vi "SimpleGit-Settings.vi"(11 "path":path) -> ()   [LabVIEW 2017]
uses:
  <vilib>/Hampel Software Engineering/Git API/Git API/GIT-api.lvclass
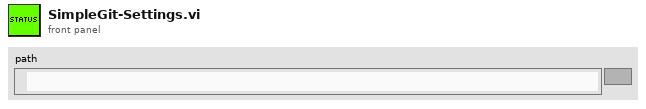
[diagram p1: front panel]
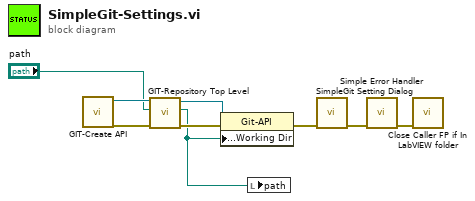
[diagram p0: block diagram]
diagram:
  n1 = call <vilib>:"GIT-Create API.vi"() -> ("error out"=w6:errorcluster, "git-api out"=w7:refnum<class "GIT-api.lvclass">)  [unwired: 10 in]
  n2 = call <vilib>:"GIT-Repository Top Level.vi"("error in"=w6, "Current Path"="path", "git-api in"=w7) -> ("error out"=w9:errorcluster, "Repo Top Level Path"=w3:path, "git-api out"=w8:refnum<class "GIT-api.lvclass">)  [unwired: 6 in]
  n3 = property class="Git-API"(reference=w8, error in=w9, "Accessors:Working Dir"=w3) -> (error out=w2:errorcluster)  [unwired: 1 out]
  n4 = local write "path"(w3) -> ()
  n5 = call "SimpleGit Setting Dialog.vi"("error in"=w2) -> ("error out"=w1:errorcluster)  [unwired: 10 in]
  n6 = call <vilib>:"Simple Error Handler.vi"("error in (no error)"=w1) -> ("error out"=w4:errorcluster)  [unwired: 4 in, 4 out]
  n7 = call "Close Caller FP if In LabVIEW folder.vi"("error in (no error)"=w4) -> ()  [unwired: 10 in, 1 out]
